vi "Read name_pos.vi"(8 "error in (no error)":errorcluster, 11 "Optics in":refnum<class "Optics.lvclass">) -> (0 "error out":errorcluster, 2 "name_pos":string, 3 "Optics out":refnum<class "Optics.lvclass">)   [LabVIEW 2018, in "Optics.lvclass"]
uses:
  Optics.lvclass
  Optics.lvclass/Optics.ctl
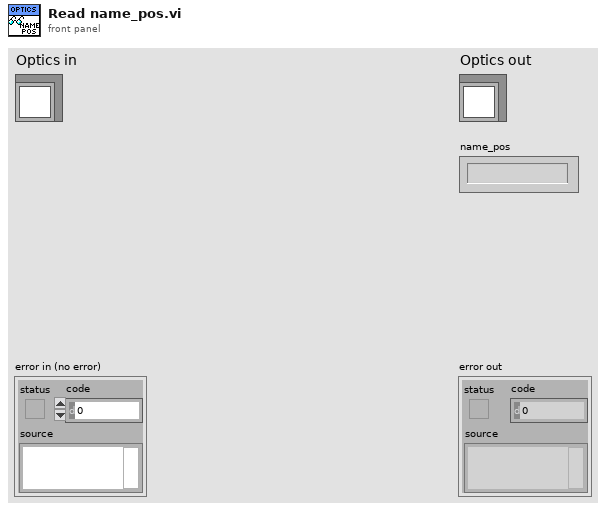
[diagram p1: front panel]
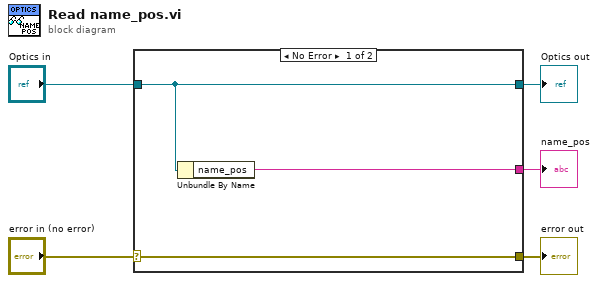
[diagram p0: block diagram]
diagram:
  n1 = case shown="No Error" "error in (no error)" {
    selector: "error in (no error)" -> [w8 w9]
    tunnel: [w8 w9] -> w4
    tunnel: [w7 w10] -> w2
    tunnel: "Optics in" -> [w7 w10]
    tunnel: [w6 _] -> w1
    frame No Error {
      n2 = Unbundle By Name(w7) -> ("name_pos"=w6:string)
    }
    frame Error {
    }
  }
  "error out" <- w4
  "Optics out" <- w2
  "name_pos" <- w1
